vi "setDefaultServerB.vi"(8 "error in (no error)":errorcluster, 11 "TcpServer.lvclass":refnum<class "TcpServer.lvclass">) -> (0 "error out":errorcluster, 3 "tcpServer out":refnum<class "TcpServer.lvclass">)   [LabVIEW 2018]
doc: "Configure the TCP/IP server B in order to run the unit test."
uses:
  src/TcpServer/TcpServer.lvclass
  src/TcpServer/configServerTypeDef.ctl
  src/TcpServerTel/typedef/enqueueOptionsTypeDef.ctl
  src/TcpServerTel/TcpServerTel.lvclass
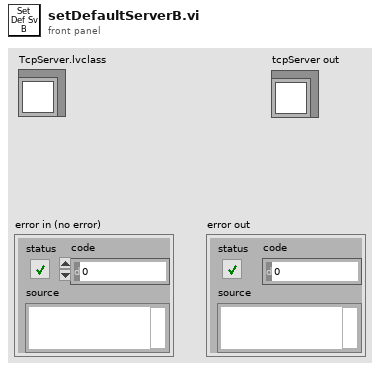
[diagram p1: front panel]
types:
  T1 = typedef "TcpServer.lvclass/configServerTypeDef.ctl" = cluster{"cmdServerPort":u16, "telServerPort":u16, "timeoutServerInMs":i32, "serverBytesToRead":i32, "maxSizeQueueTcpClientFromDds":i32, "EnqueueOptions":T2, "timeoutQueueTcpClientFromDds (ms)":i32, "maxSizeQueueTcpClient":i32, "timeoutInMs":i32}
  T2 = typedef "TcpServerTel.lvclass/enqueueOptionsTypeDef.ctl" = enum16{"lossy enqueue", "normal enqueue"}
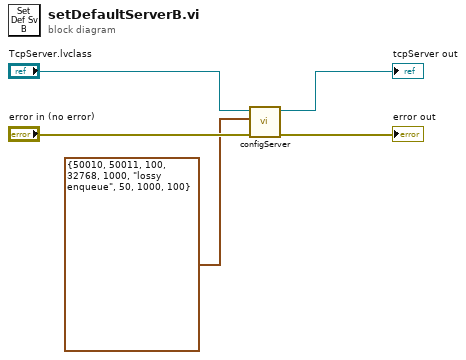
[diagram p0: block diagram]
diagram:
  n1 = call "configServer.vi"("error in (no error)"="error in (no error)", "ServerConfiguration"=T1 {"cmdServerPort"=50010, "telServerPort"=50011, "timeoutServerInMs"=100, "serverBytesToRead"=32768, "maxSizeQueueTcpClientFromDds"=1000, "EnqueueOptions"=enum."lossy enqueue", "timeoutQueueTcpClientFromDds (ms)"=50, "maxSizeQueueTcpClient"=1000, "timeoutInMs"=100}, "tcpServer in"="TcpServer.lvclass") -> ("error out"=→"error out":errorcluster, "tcpServer out"=→"tcpServer out":refnum<class "TcpServer.lvclass">)  [unwired: 7 in]
